vi "Update Tree.vi"(4 "Path Filter":string, 6 "Name Filter":string, 8 "Linker Info":T2(array[cluster]), 9 "Index Map":map{string, i32}(c390), 10 "Item":string, 11 "Tree In":refnum<vi>) -> ()   [LabVIEW 2020, in "Linker Info.lvlib"]
uses:
  Linker Info.lvlib
  <vilib>/Utility/lvfile.llb/LVFileType.ctl
  Tree Item.ctl
  <vilib>/Utility/lvfile.llb/NI_FileType.lvlib
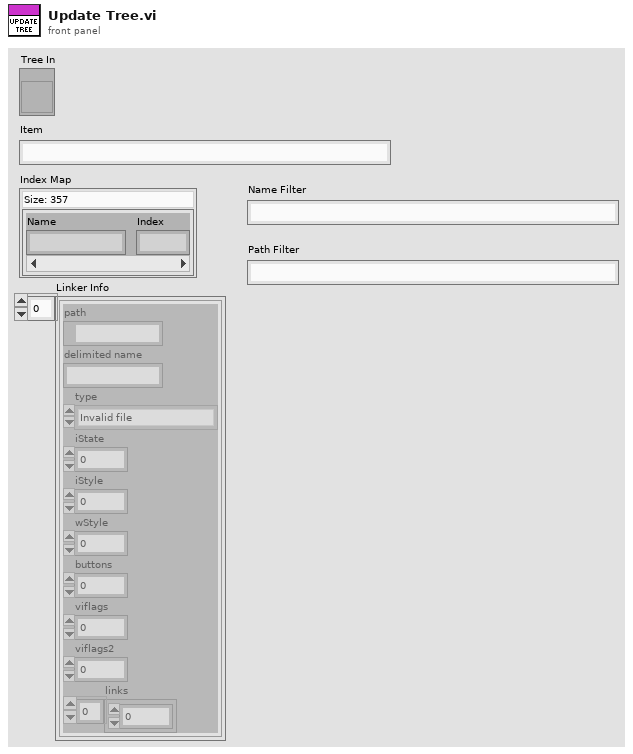
[diagram p1: front panel]
types:
  T1 = typedef "NI_FileType.lvlib/LVFileType.ctl" = enum32{"Invalid file", "Unknown type", "Instrument", "Control", "Polymorphic VI", "Project", "Library", "LVClass", "XControl", "XNode", "Shared library", ".NET assembly", "ActiveX interface", "CIN", "Run-time menu", "Palette menu", "Help file", "LLB", "XNode Edit Dependency", "Class Private Data Control", "Statechart", "MathScript .m file", "Ladder Diagram", "LVLibp", "XNode Build Dependency"}
  T2 = cluster{"path":path, "delimited name":string, "type":T1, "iState":u32, "iStyle":u16, "wStyle":u16, "buttons":u16, "viflags":u32, "viflags2":u32, "links":u32[]}[]
  T3 = typedef "Linker Info.lvlib/Tree Item.ctl" = cluster{"Name":string, "Path":string, "Parent":i32, "Level":i32, "Included":bool}
  T4 = cluster{"path":path, "delimited name":string, "type":T1, "iState":u32, "iStyle":u16, "wStyle":u16, "buttons":u16, "viflags":u32, "viflags2":u32, "links":u32[]}
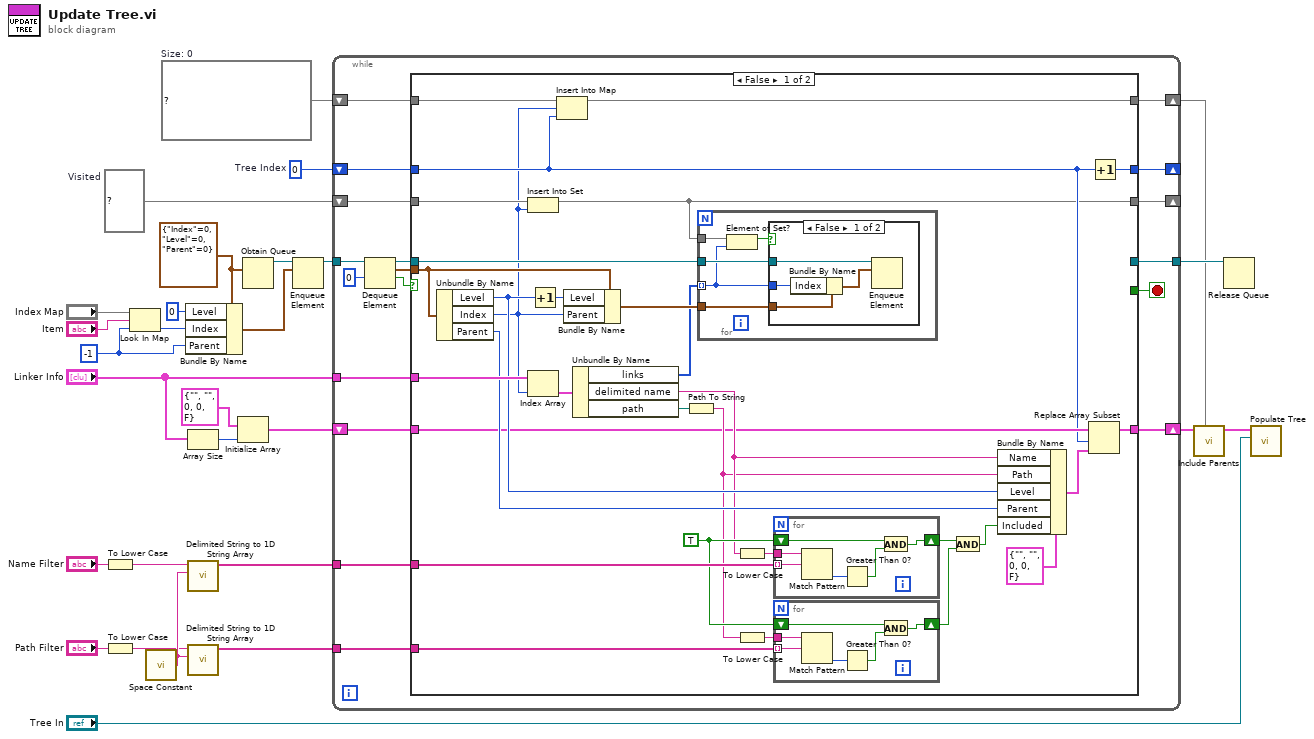
[diagram p0: block diagram]
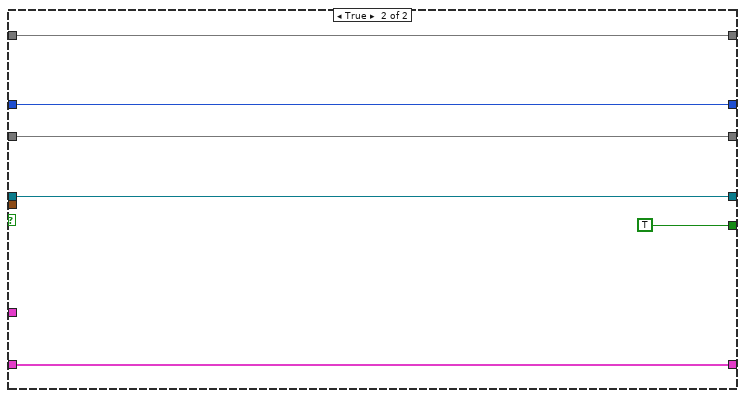
[diagram p3: hidden frame]
diagram:
  w17 = 0  # Tree Index
  w16 = map{i32, i32} {}  # Size: 0
  w15 = cluster{"Index":i32, "Level":i32, "Parent":i32} {"Index"=0, "Level"=0, "Parent"=0}
  w13 = set{i32} {}  # Visited
  w7 = -1 ("default value")
  n1 = To Lower Case(string="Name Filter") -> (all lower case string=w4:string)
  n2 = To Lower Case(string="Path Filter") -> (all lower case string=w3:string)
  n3 = Look In Map(map="Index Map", key="Item", default value=w7) -> (value=w22:i32)  [unwired: 1 out]
  n4 = call <vilib>:"Space Constant.vi"() -> ("String"=w10:string)
  n5 = Bundle By Name(cluster=w15, "Level"=u32 0, "Index"=w22, "Parent"=w7) -> (w23:cluster{"Index":i32, "Level":i32, "Parent":i32})
  n6 = Array Size(array="Linker Info") -> (size(s)=w25:i32)
  n7 = call <vilib>:"Delimited String to 1D String Array.vi"("delimiter"=w10, "delimited string"=w4) -> ("string array"=w9:string[])  [unwired: 9 in]
  n8 = call <vilib>:"Delimited String to 1D String Array.vi"("delimiter"=w10, "delimited string"=w3) -> ("string array"=w8:string[])  [unwired: 9 in]
  n9 = Initialize Array(T3 {"Name"="", "Path"="", "Parent"=0, "Level"=0, "Included"=FALSE} ("Tree item"), w25) -> (w18:T3[])
  n10 = Obtain Queue(element data type=w15) -> (queue out=w26:refnum<queue>)  [unwired: 4 in, 2 out]
  n11 = Enqueue Element(queue=w26, element=w23) -> (queue out=w21:refnum<queue>)  [unwired: 2 in, 2 out]
  n12 = while {
    tunnel: w21 -> [w46]
    tunnel: [w41] -> w20
    tunnel: "Linker Info" -> [w39]
    shift-right: [w31] -> w6
    shift-left: w18 -> [w33]
    shift-right: [w32] -> _
    shift-left: w17 -> [w38]
    shift-right: [w30] -> _
    shift-left: w13 -> [w37]
    shift-right: [w29] -> w5
    shift-left: w16 -> [w34]
    tunnel: w9 -> [w36]
    tunnel: w8 -> [w35]
    stop <- w40 stop-if-true
    n13 = Dequeue Element(queue=w46, timeout in ms (-1)=0) -> (queue out=w42:refnum<queue>, element=w43:cluster{"Index":i32, "Level":i32, "Parent":i32}, timed out?=w44:bool)  [unwired: 1 in, 1 out]
    n14 = case shown="False" w44 {
      tunnel: w43 -> [w67 _]
      tunnel: w42 -> [w68 w104]
      tunnel: [_ w104] -> w41
      tunnel: [_ TRUE] -> w40
      tunnel: w39 -> [w77 _]
      tunnel: w38 -> [w54 w99]
      tunnel: w37 -> [w75 w100]
      tunnel: w36 -> [w74 _]
      tunnel: w35 -> [w69 _]
      tunnel: w34 -> [w58 w101]
      tunnel: w33 -> [w57 w102]
      tunnel: [w55 w99] -> w32
      tunnel: [w53 w102] -> w31
      tunnel: [w51 w100] -> w30
      tunnel: [w50 w101] -> w29
      frame False {
        w71 = TRUE
        n15 = Unbundle By Name(w67) -> ("Level"=w62:i32, "Index"=w52:i32, "Parent"=w61:i32)
        n16 = Insert Into Set(10:w52, 11:w75) -> (3:w51:set{i32})  [unwired: 1 out]
        n17 = Index Array(array=w77, index=w52) -> (element=w76:T4)
        n18 = Increment(x=w62) -> (x+1=w66:i32)
        n19 = Insert Into Map(map in=w58, key=w52, value=w54) -> (map out=w50:map{i32, i32})  [unwired: 2 out]
        n20 = Bundle By Name(cluster=w67, "Level"=w66, "Parent"=w52) -> (w65:cluster{"Index":i32, "Level":i32, "Parent":i32})
        n21 = Unbundle By Name(w76) -> ("links"=w47:u32[], "delimited name"=w60:string, "path"=w70:path)
        n22 = Path To String(path=w70) -> (string=w59:string)
        n23 = for {
          tunnel: w68 -> [w81]
          tunnel: w47 -> [w78] mode=indexing
          tunnel: w51 -> [w82]
          tunnel: w65 -> [w79]
          n24 = Element of Set?(10:w78, 11:w82) -> (3:w80:bool)
          n25 = case shown="False" w80 {
            tunnel: w81 -> [w84 _]
            tunnel: w79 -> [w86 _]
            tunnel: w78 -> [w85 _]
            frame False {
              n26 = Bundle By Name(cluster=w86, "Index"=w85) -> (w83:cluster{"Index":i32, "Level":i32, "Parent":i32})
              n27 = Enqueue Element(queue=w84, element=w83) -> ()  [unwired: 2 in, 3 out]
            }
            frame True {
            }
          }
        }
        n28 = To Lower Case(string=w60) -> (all lower case string=w49:string)
        n29 = To Lower Case(string=w59) -> (all lower case string=w48:string)
        n30 = for {
          tunnel: w74 -> [w97] mode=indexing
          tunnel: w49 -> [w98]
          shift-right: [w93] -> w73
          shift-left: w71 -> [w95]
          n31 = Match Pattern(string=w98, regular expression=w97) -> (offset past match=w96:i32)  [unwired: 1 in, 3 out]
          n32 = Greater Than 0?(x=w96) -> (x > 0?=w94:bool)
          n33 = And(x=w95, y=w94) -> (x .and. y?=w93:bool)
        }
        n34 = for {
          tunnel: w69 -> [w91] mode=indexing
          tunnel: w48 -> [w92]
          shift-right: [w87] -> w72
          shift-left: w71 -> [w89]
          n35 = Match Pattern(string=w92, regular expression=w91) -> (offset past match=w90:i32)  [unwired: 1 in, 3 out]
          n36 = Greater Than 0?(x=w90) -> (x > 0?=w88:bool)
          n37 = And(x=w89, y=w88) -> (x .and. y?=w87:bool)
        }
        n38 = And(x=w73, y=w72) -> (x .and. y?=w63:bool)
        n39 = Bundle By Name(cluster=T3 {"Name"="", "Path"="", "Parent"=0, "Level"=0, "Included"=FALSE} ("Tree item"), "Name"=w60, "Path"=w59, "Level"=w62, "Parent"=w61, "Included"=w63) -> (w56:T3)
        n40 = Replace Array Subset(array=w57, new element=w56, index=w54) -> (w53:T3[])
        n41 = Increment(x=w54) -> (x+1=w55:i32)
      }
      frame True {
      }
    }
  }
  n42 = call "Include Parents.vi"("Linker Tree Map"=w5, "Tree"=w6) -> ("Updated Tree"=w2:T3[])  [unwired: 9 in]
  n43 = Release Queue(queue=w20) -> ()  [unwired: 2 in, 3 out]
  n44 = call "Populate Tree.vi"("Tree In"="Tree In", "Tree"=w2) -> ()  [unwired: 10 in]
